vi "arrayshift_I16.vi"(3 "NewArray":i16[][](array[numeric])=[[6], [7]], 4 "IndexIn":i32 min=0 step=1, 5 "SaveArray":i16[][](array[numeric])=[[0, 2, 4], [1, 3, 5]]) -> (0 "Too Big":bool, 1 "IndexOut":i32, 2 "OutArray":i16[][](array[numeric]))   [LabVIEW 2018]
uses:
  D:/LabVIEW/LabVIEWProjects/dlcTAF/dlcTAF1.1/SubVIs/64bitC_code/arrayshift_I16_C/bin/Debug/arrayshiftI16.dll
panel:
  out "NNew":i32
  out "NData":i32
  out "NChan":i32
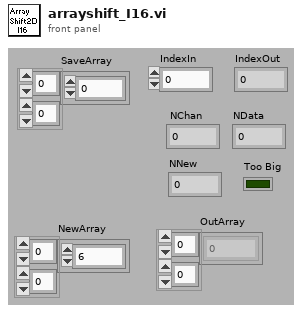
[diagram p1: front panel]
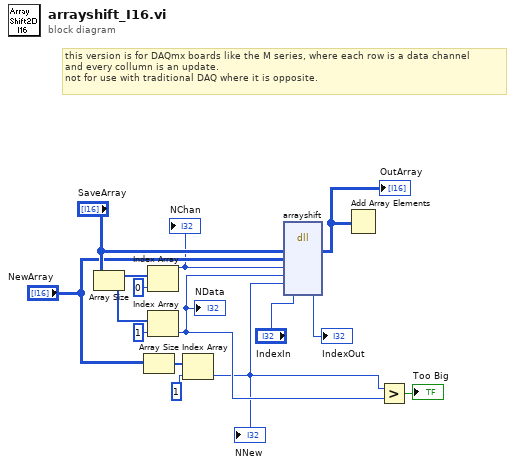
[diagram p0: block diagram]
diagram:
  # "this version is for DAQmx boards like the M series, where each row is a data channel\nand every collumn is an update.\nnot for use with traditional DAQ where it is opposite."
  n1 = Array Size(array="SaveArray") -> (size(s)=w14:i32[])
  n2 = Array Size(array="NewArray") -> (size(s)=w9:i32[])
  n3 = Index Array(array=w14, index=0 ("Index")) -> (element=w5:i32)
  "NChan" <- w5
  n4 = Index Array(array=w14, index=1 ("Index")) -> (element=w4:i32)
  "NData" <- w4
  n5 = Index Array(array=w9, index=1 ("Index")) -> (element=w3:i32)
  "NNew" <- w3
  n6 = dll-call lib="D:/LabVIEW/LabVIEWProjects/dlcTAF/dlcTAF1.1/SubVIs/64bitC_code/arrayshift_I16_C/bin/Debug/arrayshiftI16.dll" fn="arrayshift"("SaveArray"="SaveArray", "NewArray"="NewArray", "NChan"=w5, "NData"=w4, "NNew"=w3, "Index"="IndexIn") -> ("SaveArray"=w6:i16[][], "Index"=→"IndexOut":i32)  [unwired: 8 in, 2 out]
  "OutArray" <- w6
  n7 = Add Array Elements(numeric array=w6) -> ()  [unwired: 1 out]
  n8 = Greater?(x=w3, y=w4) -> (0:→"Too Big":bool)
